vi "TDS_GetConfigurationFilesList.vi"(8 "error in (no error)":errorcluster, 11 "VI Server Cluster":T1={"Refs"=[], "Labels"=["Label", "Size", "Font", "Heght", "Width", "Ledding Denominator", "Ledding Nominator", "Label Number", "Microstep Resolution", "X", "Y", "Z", "Italic?", "Underlined?"], "VI Ref"=refnum}) -> (0 "error out":errorcluster, 3 "VI Server ClusterDUP":T1={"Refs"=[], "Labels"=["Label", "Size", "Font", "Heght", "Width", "Ledding Denominator", "Ledding Nominator", "Label Number", "Microstep Resolution", "X", "Y", "Z", "Italic?", "Underlined?"], "VI Ref"=refnum})   [LabVIEW 2020]
uses:
  NA-E5071B/E5071B.llb/Labels&Control References.ctl
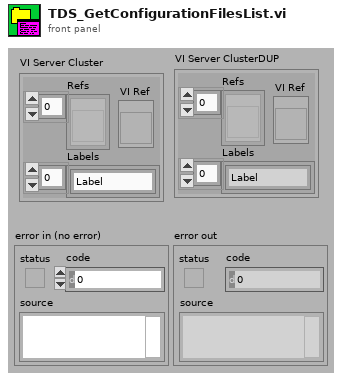
[diagram p1: front panel]
types:
  T1 = typedef "Labels&Control References.ctl" = cluster{"Refs":refnum<vi>[], "Labels":string[], "VI Ref":refnum<vi>}
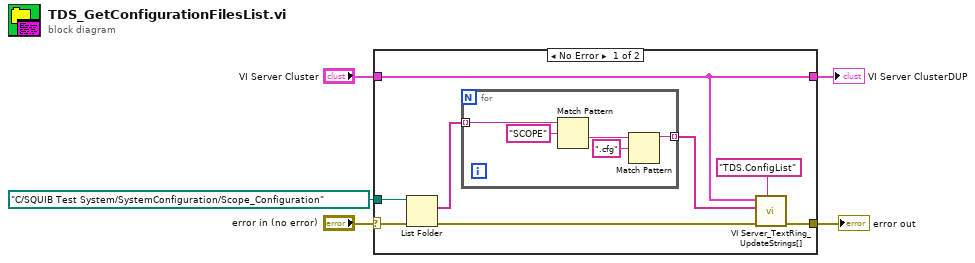
[diagram p0: block diagram]
diagram:
  n1 = case shown="No Error" "error in (no error)" {
    selector: "error in (no error)" -> [w7 w19]
    tunnel: path "C:/SQUIB Test System/SystemConfiguration/Scope_Configuration" ("path") -> [w13 _]
    tunnel: [w10 w19] -> w4
    tunnel: "VI Server Cluster" -> [w6 _]
    tunnel: [w6 _] -> w1
    frame No Error {
      n2 = List Folder(path=w13, error in=w7) -> (filenames=w12:string[], error out=w11:errorcluster)  [unwired: 2 in, 2 out]
      n3 = for {
        tunnel: w12 -> [w18] mode=indexing
        tunnel: [w14] -> w9 mode=indexing
        n4 = Match Pattern(string=w18, regular expression="SCOPE") -> (after substring=w16:string)  [unwired: 1 in, 3 out]
        n5 = Match Pattern(string=w16, regular expression=".cfg") -> (before substring=w14:string)  [unwired: 1 in, 3 out]
      }
      n6 = call "VI Server_TextRing_UpdateStrings[].vi"("Label"="TDS.ConfigList", "error in"=w11, "Strings []"=w9, "VI Server Cluster"=w6) -> ("error out"=w10:errorcluster)  [unwired: 5 in, 2 out]
    }
    frame Error {
    }
  }
  "error out" <- w4
  "VI Server ClusterDUP" <- w1
